vi "2D_array_to_1D_array.vi"(4 "Linear Index":i32, 5 "2D Input Arrray":T1[][](array[typedef]) {"Table Mode"."Freq. Step (MHz)" format="%#_9g"; "Table Mode"."FinalFreq" format="%#_9g"; "Table Mode"."Initial Freq.(MHz)" format="%#_9g"; "Channel Settings"."Frequency (MHz)" format="%#_9g"}) -> (0 "Column":i32, 1 "Row":i32, 2 "1D Output array":T1[](array[typedef]) {"Table Mode"."Freq. Step (MHz)" format="%#_9g"; "Table Mode"."FinalFreq" format="%#_9g"; "Table Mode"."Initial Freq.(MHz)" format="%#_9g"; "Channel Settings"."Frequency (MHz)" format="%#_9g"})   [LabVIEW 2016]
uses:
  Controls/Synth_409b/Synth_controls.ctl
  Controls/Synth_409b/synth_channel.ctl
  Controls/Synth_409b/table_mode.ctl
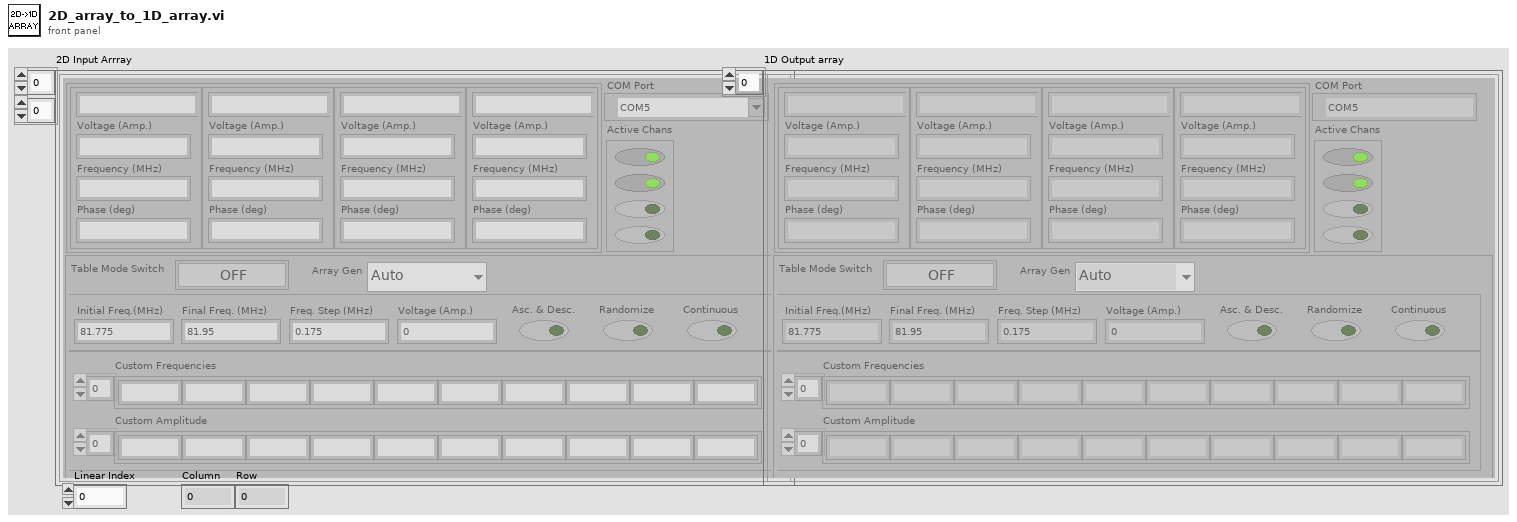
[diagram p1: front panel]
types:
  T1 = typedef "Synth_controls.ctl" = cluster{"Channel Settings":T2[], "Active Chans":bool[], "COM Port":refnum<visa-resource-name>, "Table Mode":T3}
  T2 = typedef "synth_channel.ctl" = cluster{"Voltage (Amp.) ":dbl, "Frequency (MHz)":dbl, "Phase (deg)":dbl, "Nickname":string}
  T3 = typedef "table_mode.ctl" = cluster{"Initial Freq.(MHz)":dbl, "FinalFreq":dbl, "Freq. Step (MHz)":dbl, "Voltage (Amp.)":dbl, "Asc. & Desc.":bool, "Custom Frequencies":dbl[], "Custom Amplitude":dbl[], "Table Mode Switch":bool, "Array Gen":enum16{"Auto", "Custom"}, "Randomize":bool, "Continuous":bool}
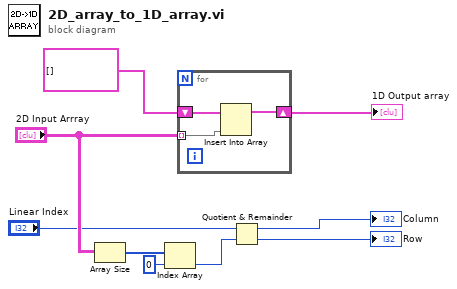
[diagram p0: block diagram]
diagram:
  n1 = Array Size(array="2D Input Arrray") -> (size(s)=w6:i32[])
  n2 = Index Array(array=w6, index=0) -> (element=w3:i32)
  n3 = for {
    tunnel: "2D Input Arrray" -> [w11] mode=indexing
    shift-right: [w10] -> w8
    shift-left: T1[] [] -> [w12]
    n4 = Insert Into Array(array=w12, new element=w11) -> (w10:T1[])  [unwired: 1 in]
  }
  "1D Output array" <- w8
  n5 = Quotient & Remainder(x="Linear Index", y=w3) -> (x-y*floor(x/y)=→"Column":i32, floor(x/y)=→"Row":i32)
